vi "GetTerminalDataType.vi"(6 "error in":errorcluster, 9 "Terminal in":refnum<class "Terminal.lvclass">) -> (0 "error out":errorcluster, 3 "Terminal out":refnum<class "Terminal.lvclass">, 4 "Data Type":variant)   [LabVIEW 2014, in "Raspberry Pi Compatible Compiler for LabVIEW.lvlib" / "Terminal.lvclass"]
uses:
  Terminal.lvclass
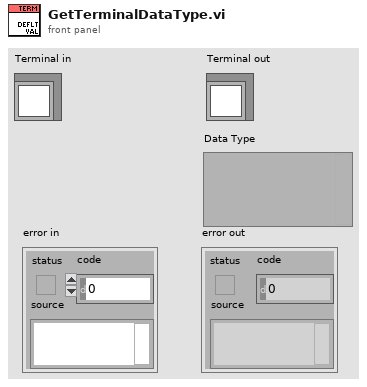
[diagram p1: front panel]
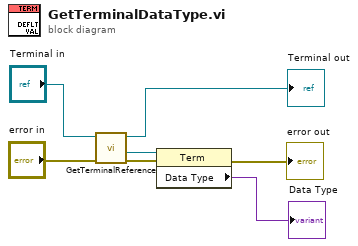
[diagram p0: block diagram]
diagram:
  n1 = call "GetTerminalReference.vi"("error in"="error in", "Terminal in"="Terminal in") -> ("error out"=w3:errorcluster, "reference"=w4:refnum<vi>, "Terminal out"=→"Terminal out":refnum<class "Terminal.lvclass">)  [unwired: 7 in]
  n2 = property class="Term"(reference=w4, error in=w3) -> (error out=→"error out":errorcluster, "Data Type"=→"Data Type":variant)  [unwired: 1 out]
